vi "LB_ItemName.vi"(11 "error in (no error)":errorcluster) -> (15 "error out":errorcluster)   [LabVIEW 2016, in "DronaTest.lvlib"]
uses:
  DronaTest.lvlib
  APIs/Stimulus/ControlValue/SetValueAuto.vi
  APIs/Stimulus/ControlValue/Controls/Listbox/SetValueByItemName.vi
  APIs/Assert/AssertControlValue/Equal.vi
  <vilib>/addons/_JKI Toolkits/Caraya/classes/Assert/Assert Equal Value_Variant.vi
  APIs/Stimulus/VI/CloseVI.vi
  <vilib>/addons/_JKI Toolkits/Caraya/classes/Test/Test.lvclass
  Drona.lvlib
  <vilib>/SLL Toolkit/SLL Debug/SLL Debug.lvlib
  APIs/Assert/AssertControlValue/AssertControlValue.lvlib
  APIs/Stimulus/ControlValue/ControlValue.lvlib
  APIs/Stimulus/VI/VI.lvlib
  <vilib>/addons/_JKI Toolkits/Caraya/classes/Assert/Assert.lvclass
  APIs/Stimulus/ControlValue/Controls/Listbox/StimulusListbox.lvlib
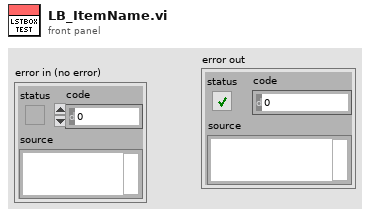
[diagram p1: front panel]
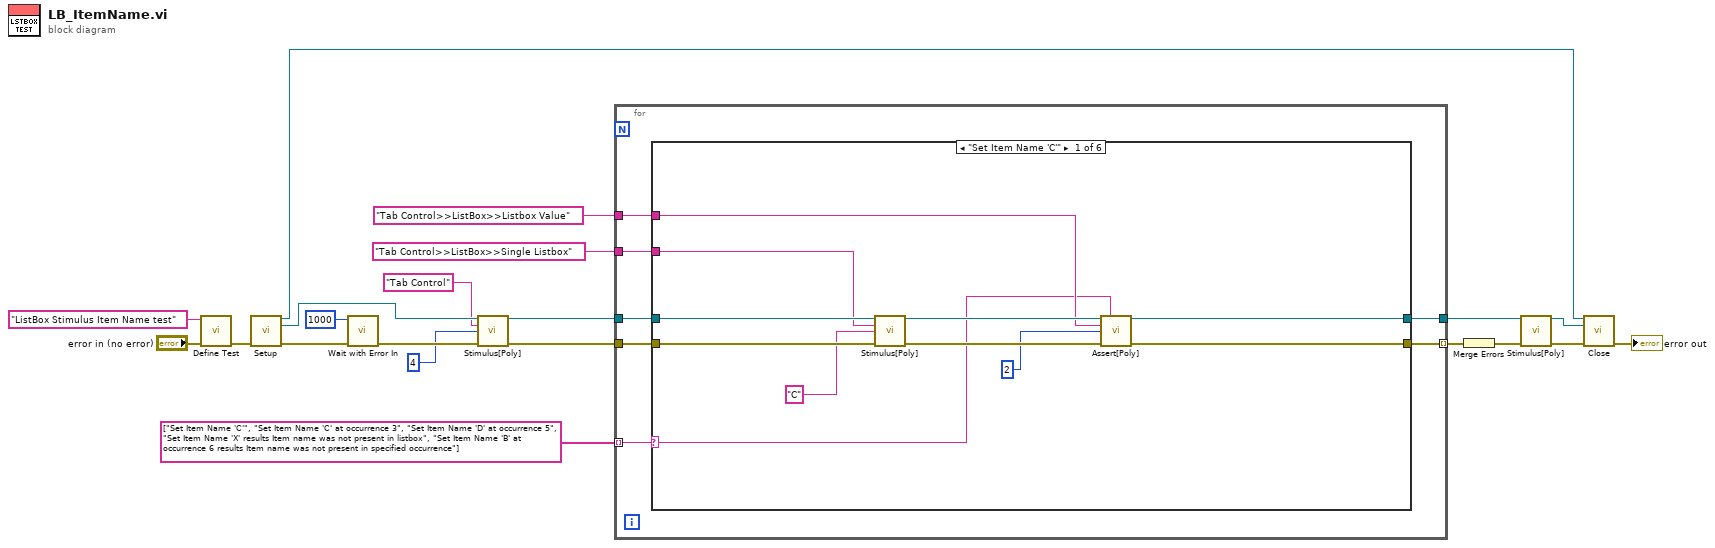
[diagram p0: block diagram]
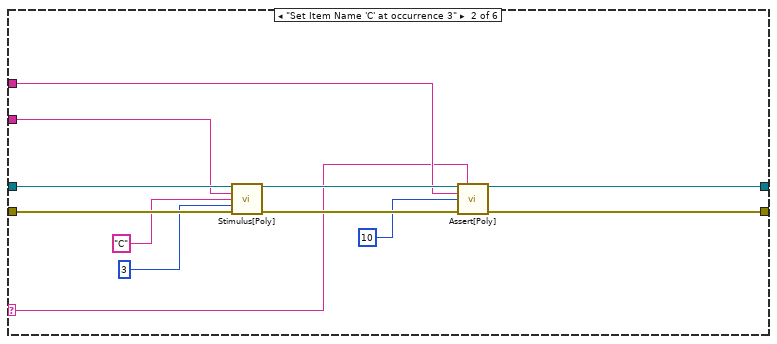
[diagram p2: hidden frame]
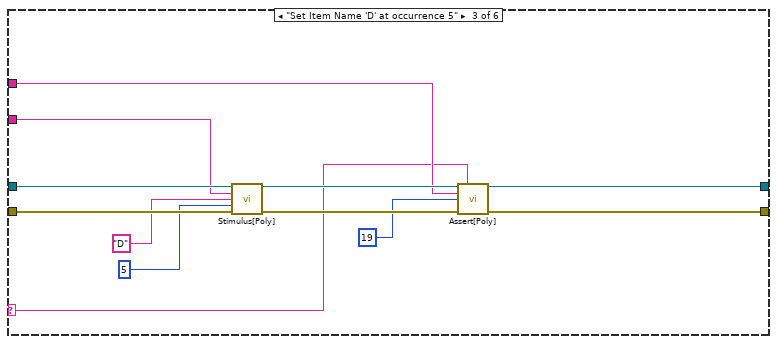
[diagram p3: hidden frame]
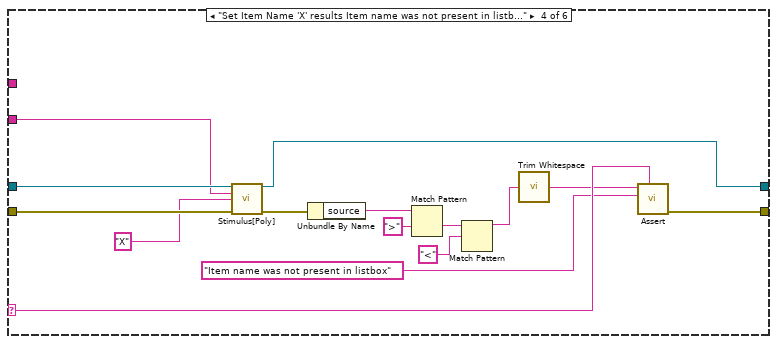
[diagram p4: hidden frame]
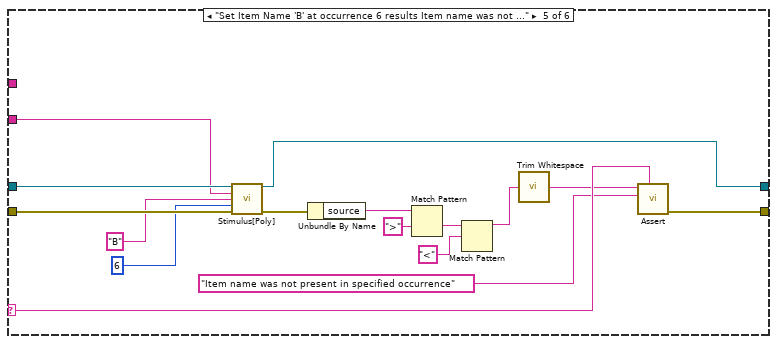
[diagram p5: hidden frame]
diagram:
  n1 = call <vilib>:"Define Test.vi"("error in (no error)"="error in (no error)", "Label (VI Title)"="ListBox Stimulus Item Name test") -> ("error out"=w20:errorcluster)  [unwired: 9 in]
  n2 = call "Setup.vi"("error in"=w20) -> ("Application Ref"=w7:refnum<vi>, "VI Reference Out"=w14:refnum<vi>, "error out"=w19:errorcluster)  [unwired: 12 in]
  n3 = call <vilib>:"Wait with Error In.vi"("error in (no error)"=w19, "milliseconds to wait"=u32 1000) -> ("error out"=w16:errorcluster)  [unwired: 9 in]
  n4 = call-poly "Stimulus[Poly].vi"("VI Reference In"=w14, "Control Path"="Tab Control", "Value (Signaling)"=4, "error in"=w16) -> ("VI Reference Out"=w10:refnum<vi>, "error out"=w15:errorcluster)  [unwired: 10 in]
  n5 = for {
    tunnel: w10 -> [w27]
    tunnel: "Tab Control>>ListBox>>Single Listbox" ("Control Path") -> [w26]
    tunnel: "Tab Control>>ListBox>>Listbox Value" ("Control Path") -> [w25]
    tunnel: string[] ["Set Item Name 'C'", "Set Item Name 'C' at occurrence 3", "Set Item Name 'D' at occurrence 5", "Set Item Name 'X' results Item name was not present in listbox", "Set Item Name 'B' at occurrence 6 results Item name was not present in specified occurrence"] -> [w23] mode=indexing
    tunnel: [w22] -> w3
    tunnel: w15 -> [w28]
    tunnel: [w24] -> w2 mode=indexing
    n6 = case shown="\"Set Item Name 'C'\"" w23 {
      selector: w23 -> [w31 w43 w55 w74 w90 _]
      tunnel: w28 -> [w39 w51 w63 w78 w94 w96]
      tunnel: w27 -> [w38 w50 w62 w77 w93 w95]
      tunnel: w26 -> [w35 w47 w59 w76 w92 _]
      tunnel: w25 -> [w34 w46 w58 _ _ _]
      tunnel: [w33 w45 w57 w75 w91 w96] -> w24
      tunnel: [w32 w44 w56 w73 w89 w95] -> w22
      frame "Set Item Name 'C'" {
        n7 = call-poly "Stimulus[Poly].vi"("VI Reference In"=w38, "Control Path"=w35, "Item Name"="C", "Error In"=w39) -> ("VI Reference Out"=w36:refnum<vi>, "Error Out"=w37:errorcluster)  [unwired: 10 in]
        n8 = call-poly "Assert[Poly].vi"("VI Reference In"=w36, "Test Label"=w31, "Control Path"=w34, "Control Value"=2, "Error In"=w37) -> ("VI Reference Out"=w32:refnum<vi>, "Error Out"=w33:errorcluster)  [unwired: 8 in, 1 out]
      }
      frame "Set Item Name 'C' at occurrence 3" {
        n9 = call-poly "Stimulus[Poly].vi"("VI Reference In"=w50, "Control Path"=w47, "Item Name"="C", "Occurrence"=3, "Error In"=w51) -> ("VI Reference Out"=w48:refnum<vi>, "Error Out"=w49:errorcluster)  [unwired: 9 in]
        n10 = call-poly "Assert[Poly].vi"("VI Reference In"=w48, "Test Label"=w43, "Control Path"=w46, "Control Value"=10, "Error In"=w49) -> ("VI Reference Out"=w44:refnum<vi>, "Error Out"=w45:errorcluster)  [unwired: 8 in, 1 out]
      }
      frame "Set Item Name 'D' at occurrence 5" {
        n11 = call-poly "Stimulus[Poly].vi"("VI Reference In"=w62, "Control Path"=w59, "Item Name"="D", "Occurrence"=5, "Error In"=w63) -> ("VI Reference Out"=w60:refnum<vi>, "Error Out"=w61:errorcluster)  [unwired: 9 in]
        n12 = call-poly "Assert[Poly].vi"("VI Reference In"=w60, "Test Label"=w55, "Control Path"=w58, "Control Value"=19, "Error In"=w61) -> ("VI Reference Out"=w56:refnum<vi>, "Error Out"=w57:errorcluster)  [unwired: 8 in, 1 out]
      }
      frame "Set Item Name 'X' results Item name was not present in listbox" {
        n13 = call-poly "Stimulus[Poly].vi"("VI Reference In"=w77, "Control Path"=w76, "Item Name"="X", "Error In"=w78) -> ("VI Reference Out"=w73:refnum<vi>, "Error Out"=w71:errorcluster)  [unwired: 10 in]
        n14 = Unbundle By Name(w71) -> ("source"=w69:string)
        n15 = Match Pattern(string=w69, regular expression=">") -> (after substring=w67:string)  [unwired: 1 in, 3 out]
        n16 = Match Pattern(string=w67, regular expression="<") -> (before substring=w65:string)  [unwired: 1 in, 3 out]
        n17 = call <vilib>:"Trim Whitespace.vi"("string"=w65) -> ("trimmed string"=w64:string)  [unwired: 1 in]
        n18 = call-poly <vilib>:"Assert.vi"("Label"=w74, "Y"="Item name was not present in listbox", "X"=w64) -> ("error out"=w75:errorcluster)  [unwired: 8 in]
      }
      frame "Set Item Name 'B' at occurrence 6 results Item name was not present in specified occurrence" {
        n19 = call-poly "Stimulus[Poly].vi"("VI Reference In"=w93, "Control Path"=w92, "Item Name"="B", "Occurrence"=6, "Error In"=w94) -> ("VI Reference Out"=w89:refnum<vi>, "Error Out"=w87:errorcluster)  [unwired: 9 in]
        n20 = Unbundle By Name(w87) -> ("source"=w85:string)
        n21 = Match Pattern(string=w85, regular expression=">") -> (after substring=w83:string)  [unwired: 1 in, 3 out]
        n22 = Match Pattern(string=w83, regular expression="<") -> (before substring=w81:string)  [unwired: 1 in, 3 out]
        n23 = call <vilib>:"Trim Whitespace.vi"("string"=w81) -> ("trimmed string"=w80:string)  [unwired: 1 in]
        n24 = call-poly <vilib>:"Assert.vi"("Label"=w90, "Y"="Item name was not present in specified occurrence", "X"=w80) -> ("error out"=w91:errorcluster)  [unwired: 8 in]
      }
      frame Default {
      }
    }
  }
  n25 = Merge Errors(w2) -> (w1:errorcluster)
  n26 = call-poly "Stimulus[Poly].vi"("VI Reference In"=w3, "error in"=w1) -> ("VI Reference Out"=w9:refnum<vi>, "error out"=w8:errorcluster)  [unwired: 12 in]
  n27 = call "Close.vi"("Application Ref"=w7, "VI Reference"=w9, "error in"=w8) -> ("error out"=→"error out":errorcluster)  [unwired: 12 in]
